vi "Create.vi"(8 "error in (no error)":errorcluster, 10 "Plugins":refnum<class "Plugin.lvclass">[](array[class]), 11 "Scheduler type":refnum<class "Scheduler.lvclass">) -> (0 "error out":errorcluster, 3 "Scheduler":refnum<class "Scheduler.lvclass">)   [LabVIEW 2017, in "DSF Core.lvlib" / "Scheduler.lvclass"]
uses:
  Scheduler.lvclass
  Plugin/Plugin.lvclass
  Scheduler Plugin Bundle.lvclass
  Plugin/Plugin.lvclass/Plugin.ctl
  Scheduler.lvclass/Scheduler.ctl
  Timing/Timing.lvclass
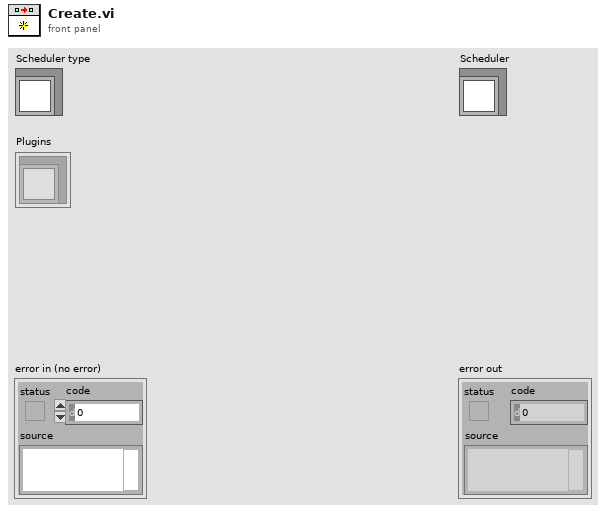
[diagram p1: front panel]
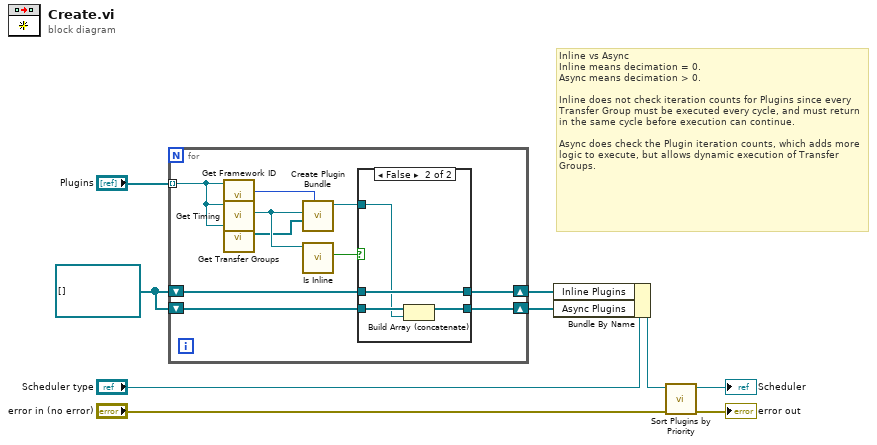
[diagram p0: block diagram]
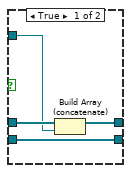
[diagram p2: hidden frame]
diagram:
  w7 = refnum<class "Scheduler Plugin Bundle.lvclass">[] [] ("Plugin Timing Group")
  # "Inline vs Async\nInline means decimation = 0.\nAsync means decimation > 0.\n\nInline does not check iteration counts for Plugins since every Transfer Group must be executed every cycle, and must return in the same cycle before execution can continue.\n\nAsync does check the Plugin iteration counts, which adds more logic to execute, but allows dynamic execution of Transfer Groups."
  n1 = for {
    tunnel: "Plugins" -> [w14] mode=indexing
    shift-right: [w18] -> w5
    shift-left: w7 -> [w19]
    shift-right: [w16] -> w6
    shift-left: w7 -> [w17]
    n2 = call "Get Framework ID.vi"("Plugin in"=w14) -> ("framework id"=w15:i32)  [unwired: 9 in, 1 out]
    n3 = call "Get Timing.vi"("Plugin in"=w14) -> ("Timing"=w13:refnum<class "Timing.lvclass">)  [unwired: 9 in, 1 out]
    n4 = call "Get Transfer Groups.vi"("Plugin in"=w14) -> ("Transfer Groups"=w10:refnum<class "Transfer Group.lvclass">[])  [unwired: 9 in, 1 out]
    n5 = call "Create Plugin Bundle.vi"("ID"=w15, "Transfer Groups"=w10, "Timing"=w13) -> ("Scheduler Plugin Bundle out"=w11:refnum<class "Scheduler Plugin Bundle.lvclass">)  [unwired: 7 in, 1 out]
    n6 = call "Is Inline.vi"("Timing in"=w13) -> ("inline?"=w12:bool)  [unwired: 9 in, 1 out]
    n7 = case shown="False" w12 {
      tunnel: w11 -> [w22 w24]
      tunnel: w19 -> [w23 w25]
      tunnel: [w21 w25] -> w18
      tunnel: w17 -> [w20 w27]
      tunnel: [w20 w26] -> w16
      frame True {
        n8 = Build Array (concatenate)(w23, w22) -> (w21:refnum<class "Scheduler Plugin Bundle.lvclass">[])
      }
      frame False {
        n9 = Build Array (concatenate)(w27, w24) -> (w26:refnum<class "Scheduler Plugin Bundle.lvclass">[])
      }
    }
  }
  n10 = Bundle By Name(cluster="Scheduler type", "Inline Plugins"=w5, "Async Plugins"=w6) -> (w4:refnum<class "Scheduler.lvclass">)
  n11 = call "Sort Plugins by Priority.vi"("error in (no error)"="error in (no error)", "Scheduler in"=w4) -> ("error out"=→"error out":errorcluster, "Scheduler out"=→"Scheduler":refnum<class "Scheduler.lvclass">)  [unwired: 8 in]
